vi "Logging Reading Cache.vi"(4 "error in (no error)":errorcluster, 5 "Mode":enum16{"Get", "Set"}(ring), 6 "Written Block":T1, 7 "refnum":refnum<file>) -> (0 "error out":errorcluster, 2 "Out":T2[](array[typedef]), 3 "refnum":refnum<file>)   [LabVIEW 2012, in "femtoRoboLib.lvlib"]
uses:
  femtoRoboLib.lvlib
  Controls/Log Entry - Converted.ctl
  Controls/Log Entry - Written Block.ctl
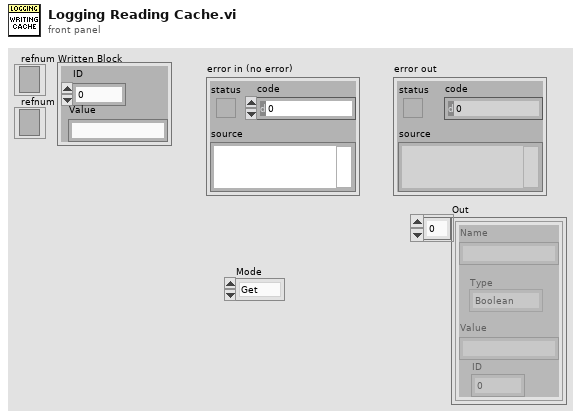
[diagram p1: front panel]
types:
  T1 = typedef "Log Entry - Written Block.ctl" = cluster{"ID":u32, "Value":string}
  T2 = typedef "femtoRoboLib.lvlib/Log Entry - Converted.ctl" = cluster{"Name":string, "Type":enum16{"Boolean", "Numeric", "String", "Boolean Array", "Numeric Array", "String Array"}, "Value":string, "ID":u32}
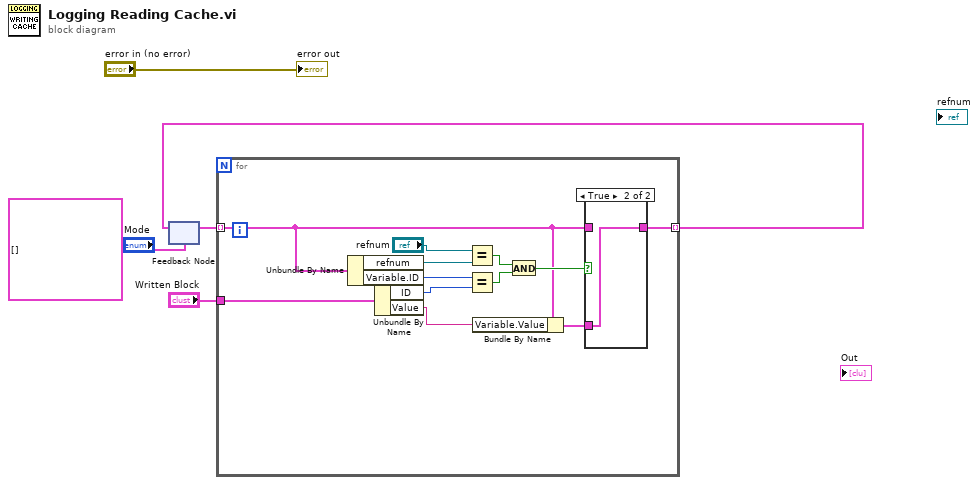
[diagram p0: block diagram]
diagram:
  n1 = feedback #1(cluster{"Variable":T2, "refnum":refnum<file>}[] []) -> (w4:cluster{"Variable":T2, "refnum":refnum<file>}[])
  n2 = for {
    tunnel: w4 -> [w7] mode=indexing
    tunnel: [w10] -> w2 mode=indexing
    tunnel: "Written Block" -> [w6]
    n3 = Unbundle By Name(w7) -> ("refnum"=w16:refnum<file>, "Variable.ID"=w15:u32)
    n4 = Unbundle By Name(w6) -> ("ID"=w14:u32, "Value"=w9:string)
    n5 = Equal?(x="refnum", y=w16) -> (x = y?=w12:bool)
    n6 = Equal?(x=w15, y=w14) -> (x = y?=w13:bool)
    n7 = Bundle By Name(cluster=w7, "Variable.Value"=w9) -> (w8:cluster{"Variable":T2, "refnum":refnum<file>})
    n8 = And(x=w12, y=w13) -> (x .and. y?=w11:bool)
    n9 = case shown="True" w11 {
      tunnel: [w18 w19] -> w10
      tunnel: w7 -> [w18 _]
      tunnel: w8 -> [_ w19]
      frame False {
      }
      frame True {
      }
    }
  }
  n10 = feedback-in #1(w2) -> ()
  "error out" <- "error in (no error)"
